vi "kf_predict.vi"(9 "Steps":sgl, 11 "KF in":T2={"A"=[], "B"=[], "H"=[], "Q"=[], "R"=[], "x"=[], "P"=[], "x lim"=[], "y lim"=[], "K"=[], "Converge count"=-1} {"K" format="%#_3g"; "y lim" format="%#_3g"; "x lim" format="%#_3g"; "P" format="%#_3g"; "H" format="%#_3g"; "x" format="%#_3g"; "Q" format="%#_3g"; "R" format="%#_3g"; "B" format="%#_3g"; "A" format="%#_3g"}) -> (2 "Predicted state":T1 caption="x" format="%#_3g")   [LabVIEW 2014]
uses:
  kalman_filter.ctl
  <vilib>/Analysis/Matrix/Datatypes/RealMatrix.ctl
  <vilib>/Analysis/baseanly.llb/Real A x B.vi
  <vilib>/Analysis/Matrix/Numeric/Add/Add - RM,RM.vi
  <vilib>/Analysis/Matrix/Numeric/Multiply/Multiply - R,RM.vi
  <vilib>/Analysis/Matrix/Numeric/Subtract/Subtract - RM,RM.vi
  <vilib>/Analysis/baseanly.llb/Real Inverse Matrix.vi
  <vilib>/Analysis/NI_AALBase.lvlib
  <vilib>/Analysis/Matrix/NI_Matrix.lvlib
panel:
  # "Predict KF state forward by specified number of time steps (may be negative.)  Conceptually this is the matrix exponent of A applied to the state, but we implement by iteration so that the state limits (x lim) can be enforced at each update.  Fractional exponents are supported by doing linear interpolation on the state."
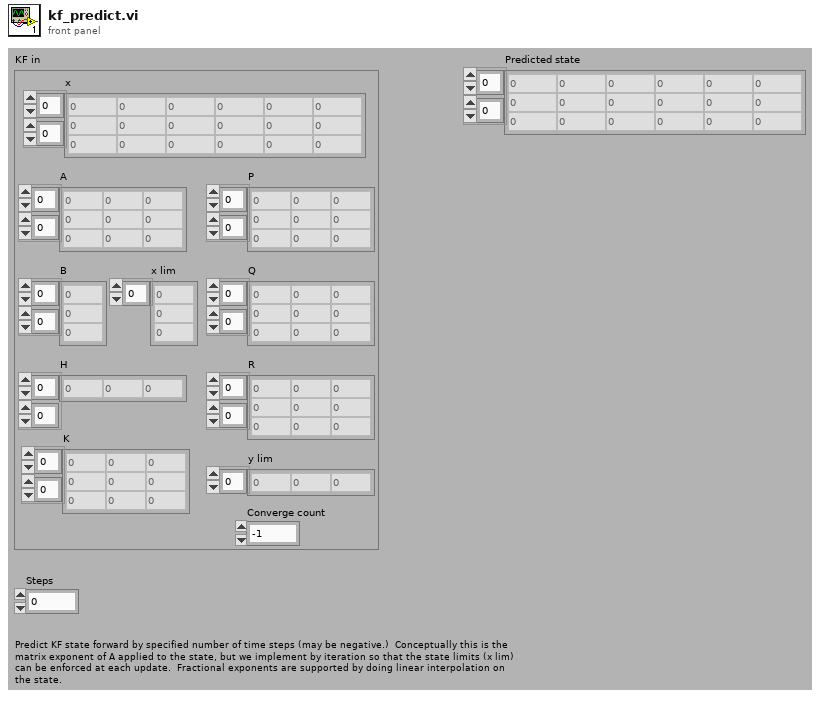
[diagram p1: front panel]
types:
  T1 = typedef "NI_Matrix.lvlib/RealMatrix.ctl" = dbl[][]
  T2 = typedef "kalman_filter.ctl" = cluster{"A":T1, "B":T1, "H":T1, "Q":T1, "R":T1, "x":T1, "P":T1, "x lim":dbl[], "y lim":dbl[], "K":T1, "Converge count":i32}
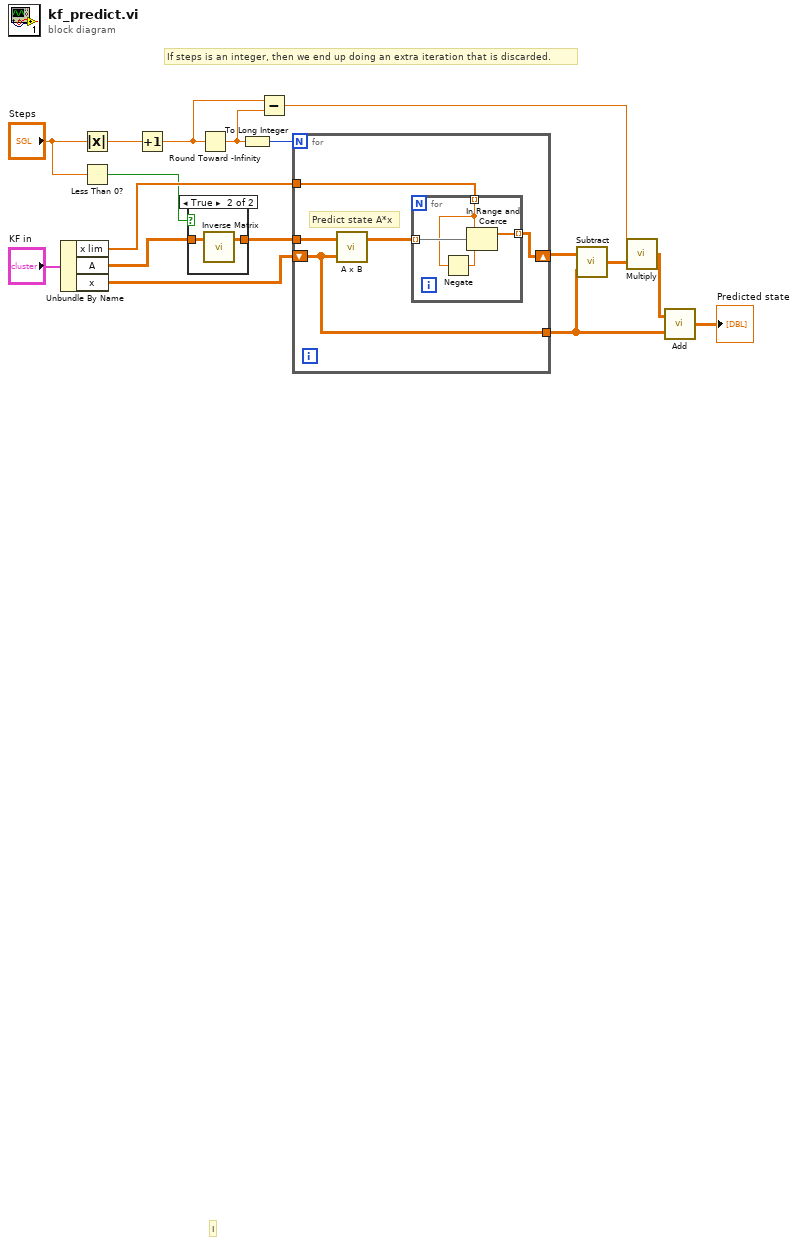
[diagram p0: block diagram]
diagram:
  # "If steps is an integer, then we end up doing an extra iteration that is discarded."
  # "I"
  n1 = Unbundle By Name("KF in") -> ("x lim"=w15:dbl[], "A"=w12:T1, "x"=w17:T1)
  n2 = Absolute Value(x="Steps") -> (abs(x)=w7:sgl)
  n3 = Less Than 0?(x="Steps") -> (x < 0?=w13:bool)
  n4 = Increment(x=w7) -> (x+1=w6:sgl)
  n5 = case shown="True" w13 {
    tunnel: w12 -> [w18 w20]
    tunnel: [w18 w19] -> w11
    frame False {
    }
    frame True {
      n6 = call-poly <vilib>:"Inverse Matrix.vi"("Input Matrix"=w20) -> ("Inverse Matrix"=w19:T1)  [unwired: 1 in, 1 out]
    }
  }
  n7 = Round Toward -Infinity(1:w6) -> (0:w9:sgl)
  n8 = To Long Integer(number=w9) -> (32bit integer=w10:i32)
  n9 = Subtract(x=w6, y=w9) -> (x-y=w5:sgl)
  n10 = for {
    N: w10 -> [_]
    tunnel: w15 -> [w24]
    tunnel: w11 -> [w25]
    shift-right: [w22] -> w3
    shift-left: w17 -> [w21]
    tunnel: [w21] -> w2
    # "Predict state A*x"
    n11 = call-poly <vilib>:"A x B.vi"("B"=w21, "A"=w25) -> ("A x B"=w23:T1)  [unwired: 1 out]
    n12 = for {
      tunnel: w23 -> [w29] mode=indexing
      tunnel: w24 -> [w28] mode=indexing
      tunnel: [w26] -> w22 mode=indexing
      n13 = Negate(x=w28) -> (-x=w27:dbl)
      n14 = In Range and Coerce(upper limit=w28, x=w29, lower limit=w27) -> (coerced(x)=w26:dbl[])  [unwired: 1 out]
    }
  }
  n15 = call-poly <vilib>:"Subtract.vi"("Real Matrix B"=w2, "Real Matrix A"=w3) -> ("A - B"=w1:T1)
  n16 = call-poly <vilib>:"Multiply.vi"("Real Matrix A"=w1, "Real Scalar c"=w5) -> ("c * A"=w8:T1)
  n17 = call-poly <vilib>:"Add.vi"("Real Matrix B"=w2, "Real Matrix A"=w8) -> ("A + B"=→"Predicted state":T1)
